vi "AMX-电源尾正面标签漏线检测参数读取.vi"(7 "error in (no error)":errorcluster caption="错误输入（无错误）", 10 "基路径":path) -> (0 "error out":errorcluster caption="错误输出", 1 "UI电源尾正面漏线参数":T2={"Rectangle"={"Left"=0, "Top"=0, "Right"=0, "Bottom"=0, "Rotation"=0.0}, "模板路径"=path "C:/Users/delluser001/Desktop/PowerLine Inspect System/Source Code/Template Program/potteryTemplete/Color.png", "Match Mode "=0, "Minimum Match Score "=800.0, "Number of Matches Requested"=1, "Rotation Angle Ranges (degrees)"=[{"Min"=-180.0, "Max"=180.0}], "Color Sensitivity "=0, "Match Offset"={"X"=0.0, "Y"=0.0}, "Color Score Weight "=500.0, "Search Strategy "=0, "Subpixel Accuracy "=FALSE, "Range (Threshold 1)"={"Lower value"=177.0, "Upper value"=255.0}} {"Rectangle"."Rotation" format="%.2f"; "Rectangle"."Left" scale=0.0..1024.0; "Rectangle"."Right" scale=0.0..1024.0; "Search Strategy" items=["Conservative", "Balance", "Aggressive", "Very Aggressive"]; "Color Sensitivity" items=["Low Sensitivity", "Medium Sensitivity", "High Sensitivity"]; "Match Mode" items=["Shift Invariant", "Rotation Invariant"]}, 2 "UI电源尾正面漏线基础参数":T3={"IsNorImage"=TRUE, "Exposure Values"=100289, "ImagePath"=path "C:/Users/hedongpo/Desktop/514-hdp/Alignment Assemble System/Test Picture/B/3.bmp"} caption="参数界面" {"Exposure Values" scale=0.0..200000.0})   [LabVIEW 2017]
uses:
  <vilib>/Utility/xml.llb/Read From XML File(string).vi
  Global System.vi
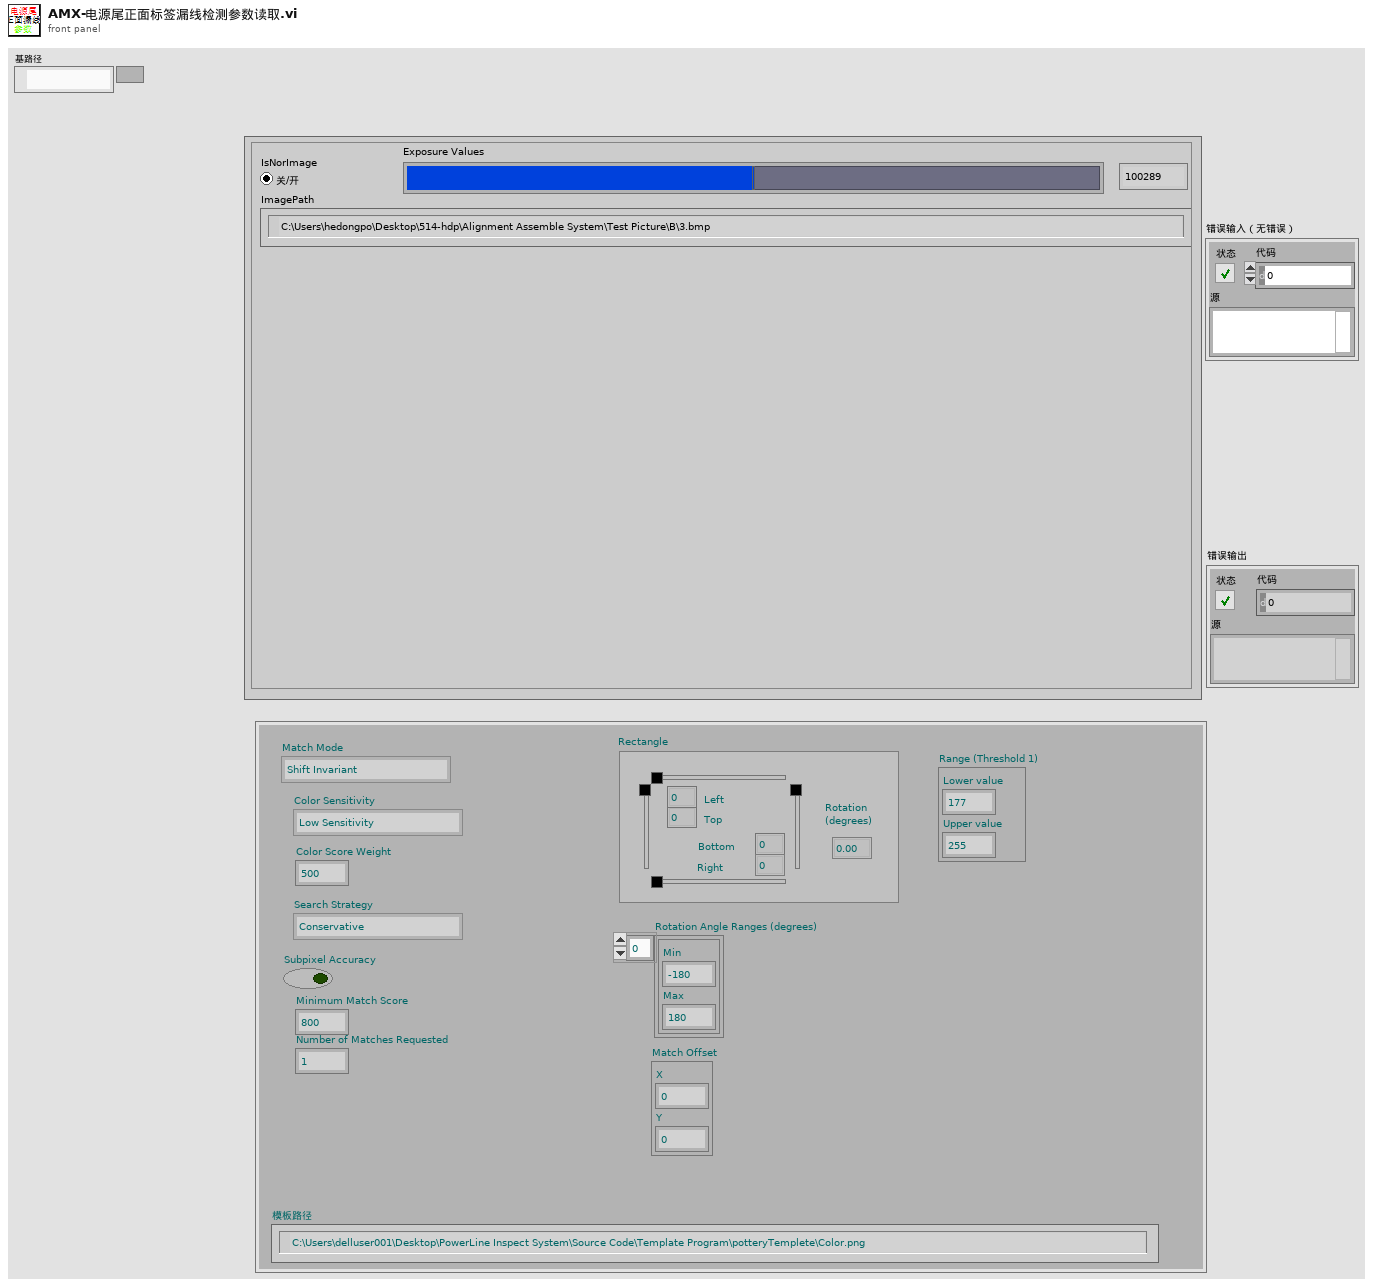
[diagram p1: front panel]
types:
  T1 = typedef "IMAQ Rectangle" = cluster{"Left":i32, "Top":i32, "Right":i32, "Bottom":i32, "Rotation":dbl}
  T2 = cluster{"Rectangle":T1, "模板路径":path, "Match Mode ":u32, "Minimum Match Score ":sgl, "Number of Matches Requested":i32, "Rotation Angle Ranges (degrees)":cluster{"Min":sgl, "Max":sgl}[], "Color Sensitivity ":u32, "Match Offset":cluster{"X":sgl, "Y":sgl}, "Color Score Weight ":sgl, "Search Strategy ":u32, "Subpixel Accuracy ":bool, "Range (Threshold 1)":cluster{"Lower value":sgl, "Upper value":sgl}}
  T3 = cluster{"IsNorImage":bool, "Exposure Values":u32, "ImagePath":path}
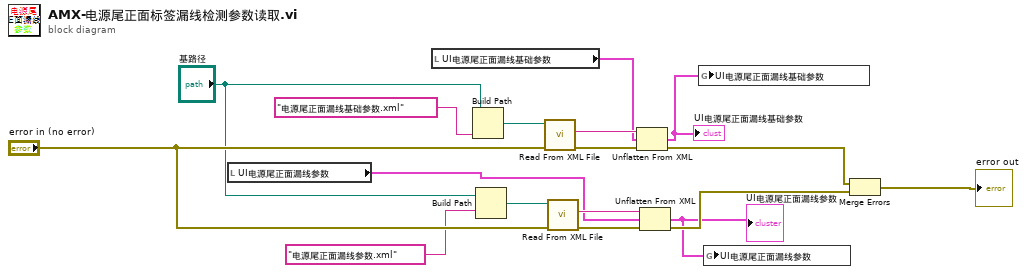
[diagram p0: block diagram]
diagram:
  n1 = local read "UI电源尾正面漏线参数"() -> (w5:T2)
  n2 = local read "UI电源尾正面漏线基础参数"() -> (w13:T3)
  n3 = Build Path(base path="基路径", name or relative path="电源尾正面漏线基础参数.xml" ("名称或相对路径")) -> (appended path=w17:path)
  n4 = Build Path(base path="基路径", name or relative path="电源尾正面漏线参数.xml" ("名称或相对路径")) -> (appended path=w14:path)
  n5 = call-poly <vilib>:"Read From XML File.vi"("error in (no error)"="error in (no error)", "XML File Path"=w17) -> ("error out"=w11:errorcluster, "XML Elements"=w16:string)  [unwired: 7 in, 1 out]
  n6 = call-poly <vilib>:"Read From XML File.vi"("error in (no error)"="error in (no error)", "XML File Path"=w14) -> ("error out"=w9:errorcluster, "XML Elements"=w15:string)  [unwired: 7 in, 1 out]
  n7 = Unflatten From XML(xml string=w16, type=w13, error in (no error)=w11) -> (value=w2:T3, error out=w10:errorcluster)
  "UI电源尾正面漏线基础参数" <- w2
  n8 = Unflatten From XML(xml string=w15, type=w5, error in (no error)=w9) -> (value=w1:T2, error out=w8:errorcluster)
  "UI电源尾正面漏线参数" <- w1
  n9 = global write "Global System.vi" "UI电源尾正面漏线基础参数"(w2) -> ()
  n10 = global write "Global System.vi" "UI电源尾正面漏线参数"(w1) -> ()
  n11 = Merge Errors(w10, w8) -> (→"error out":errorcluster)
